vi "RemoveCaliperEntry.vi"(6 "CaliperListName":string, 7 "AnalysisResult":string[][](array[string]), 9 "CaliperList":i32, 11 "CaliperEntryList":T1[](array[typedef]) {"CaliperType" items=["Distance", "Mid Point", "Perpendicular Projection", "Lines Intersection", "Angle from Horizontal", "Angle from Vertical", "Angle Defined by 3 Points", "Angle Defined by 4 Points", "Bissecting Line", "Mid Line", "Center of Mass", "Area", "Line Fit", "Circle Fit", "Ellipse Fit"]}) -> (3 "CaliperEntryList Out":T1[](array[typedef]) {"CaliperType" items=["Distance", "Mid Point", "Perpendicular Projection", "Lines Intersection", "Angle from Horizontal", "Angle from Vertical", "Angle Defined by 3 Points", "Angle Defined by 4 Points", "Bissecting Line", "Mid Line", "Center of Mass", "Area", "Line Fit", "Circle Fit", "Ellipse Fit"]})   [LabVIEW 2019]
uses:
  Controls/CaliperDataEntry.ctl
  Controls/CaliperType.ctl
  Controls/SelectionListEntry.ctl
  Controls/SelectionListEntryPointType.ctl
  Controls/CaliperResult.ctl
panel:
  out "indexes of element":i32[](array[numeric])
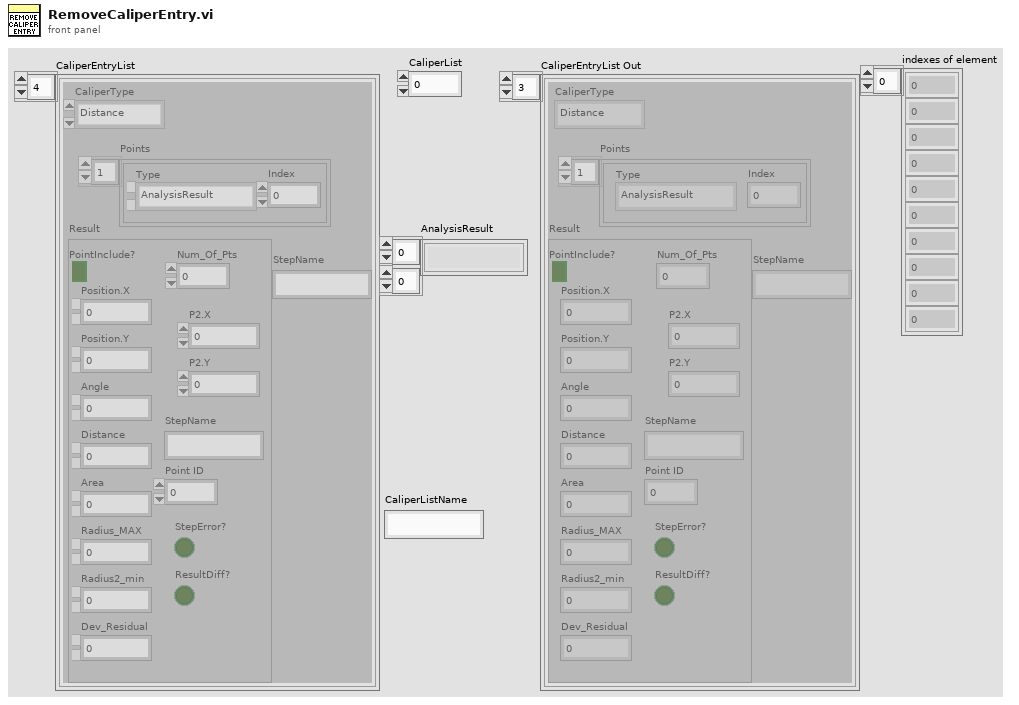
[diagram p1: front panel]
types:
  T1 = typedef "CaliperDataEntry.ctl" = cluster{"CaliperType":T2, "Points":T3[], "Result":T5, "StepName":string}
  T2 = typedef "CaliperType.ctl" = u32
  T3 = typedef "SelectionListEntry.ctl" = cluster{"Type":T4, "Index":i32}
  T4 = typedef "SelectionListEntryPointType.ctl" = enum16{"AnalysisResult", "CaliperResult"}
  T5 = typedef "CaliperResult.ctl" = cluster{"PointInclude?":bool, "Num_Of_Pts":u8, "Position.X":dbl, "Position.Y":dbl, "Angle":dbl, "Distance":dbl, "Area":dbl, "Radius_MAX":dbl, "Radius2_min":dbl, "Dev_Residual":dbl, "P2.X":dbl, "P2.Y":dbl, "StepName":string, "Point ID":u8, "StepError?":bool, "ResultDiff?":bool}
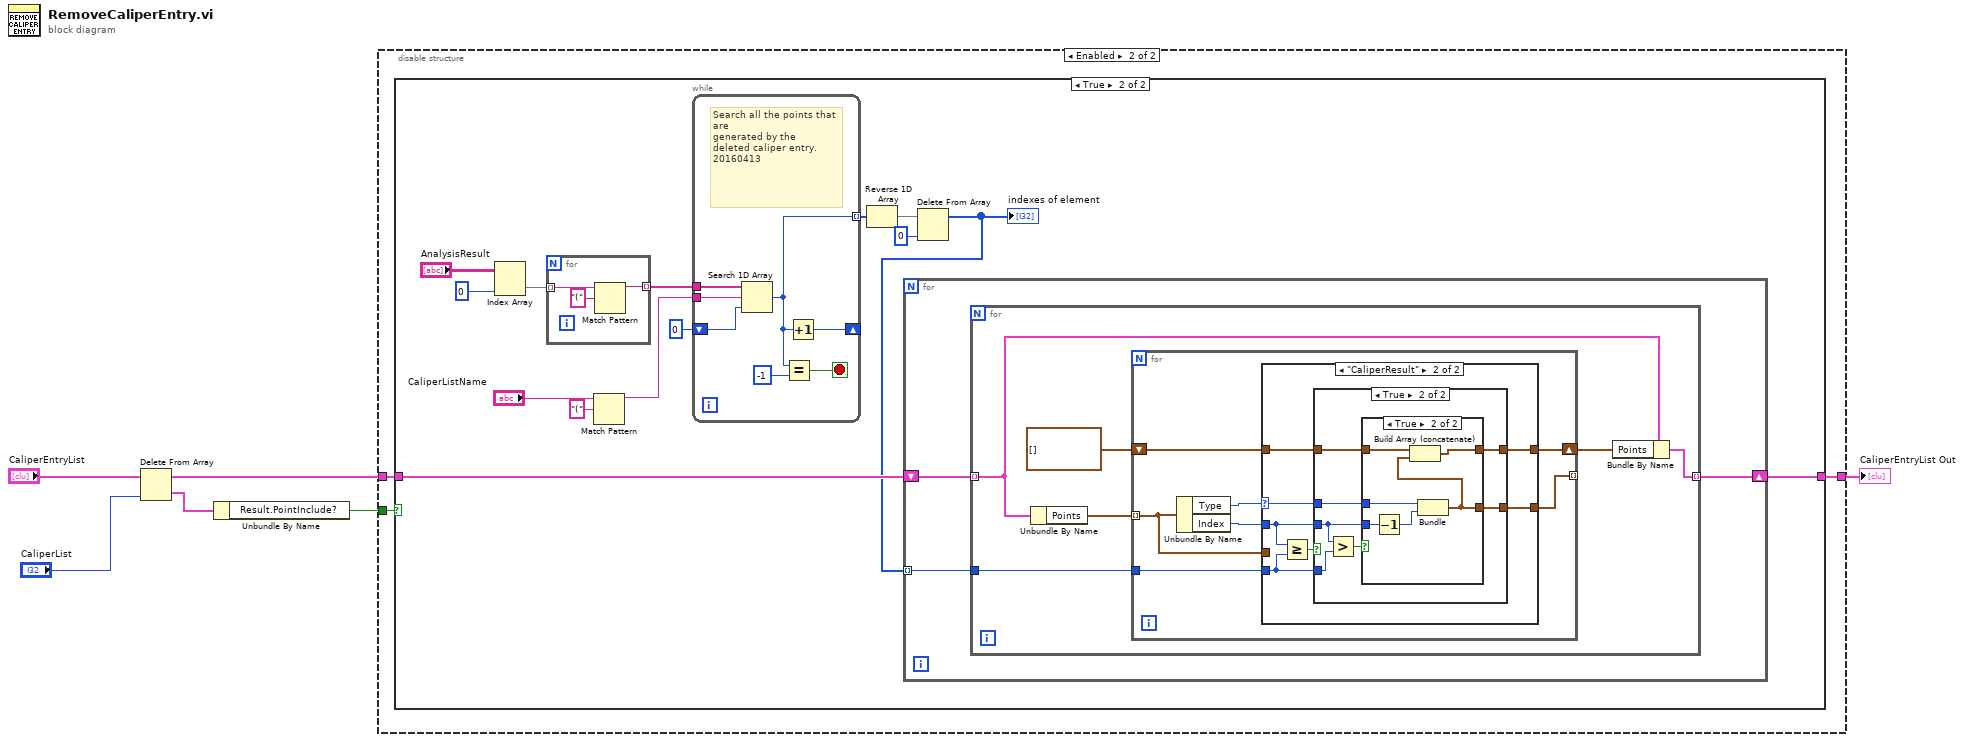
[diagram p0: block diagram]
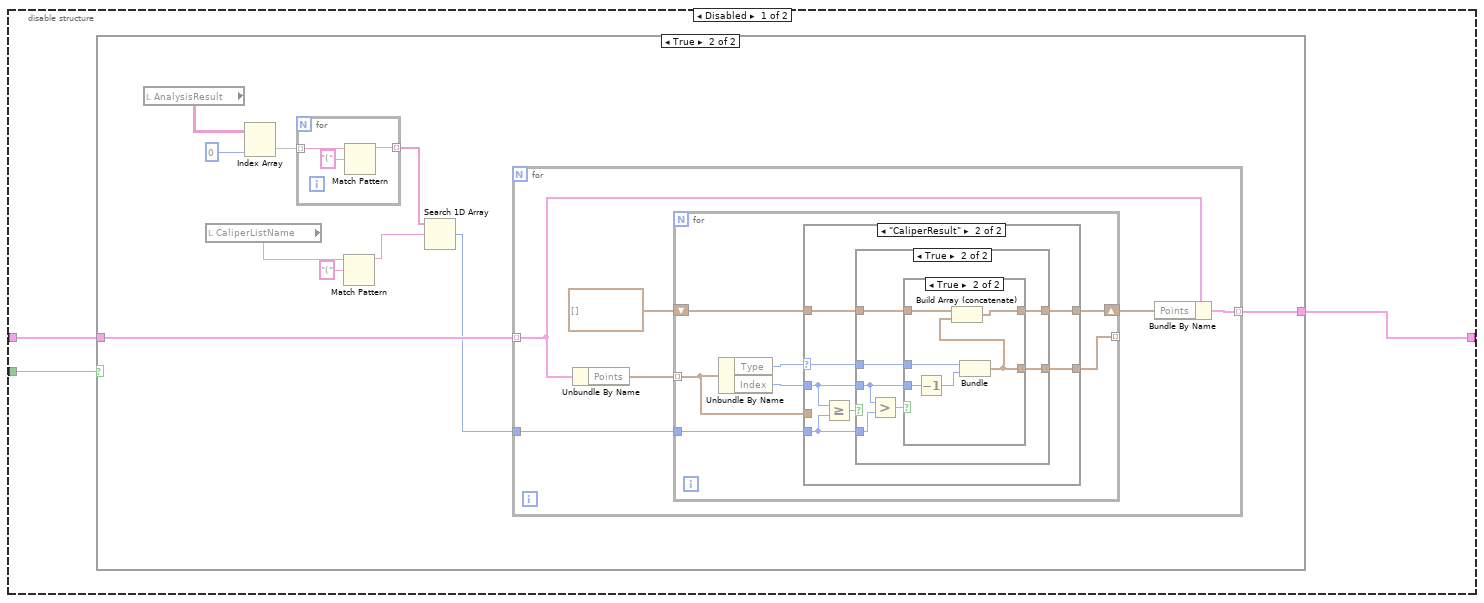
[diagram p2: hidden frame]
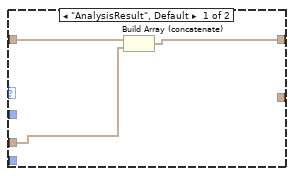
[diagram p4: hidden frame]
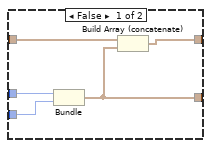
[diagram p5: hidden frame]
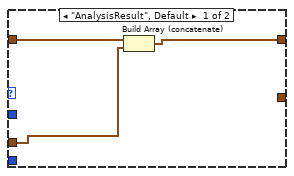
[diagram p8: hidden frame]
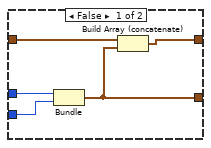
[diagram p9: hidden frame]
diagram:
  n1 = Delete From Array(array="CaliperEntryList", index="CaliperList") -> (deleted portion=w2:T1, array with subset deleted=w6:T1[])  [unwired: 1 in]
  n2 = Unbundle By Name(w2) -> ("Result.PointInclude?"=w1:bool)
  n3 = disable-structure shown="Enabled" {
    disable-tunnel: w6 -> [w9 w68]
    disable-tunnel: [w8 w67] -> w3
    disable-tunnel: w1 -> [w7 w66]
    frame Disabled {
      n4 = case shown="True" w7 {
        tunnel: w9 -> [w10 w20]
        tunnel: [w10 w19] -> w8
        frame False {
        }
        frame True {
          n5 = local read "AnalysisResult"() -> (w12:string[][])
          n6 = local read "CaliperListName"() -> (w11:string)
          n7 = Index Array(array=w12, index (col)=0 ("disabled index (col)")) -> (element=w17:string[])  [unwired: 1 in]
          n8 = for {
            tunnel: w17 -> [w23] mode=indexing
            tunnel: [w21] -> w16 mode=indexing
            n9 = Match Pattern(string=w23, regular expression="(") -> (before substring=w21:string)  [unwired: 1 in, 3 out]
          }
          n10 = Match Pattern(string=w11, regular expression="(") -> (before substring=w14:string)  [unwired: 1 in, 3 out]
          n11 = Search 1D Array(1D array=w16, element=w14) -> (index of element=w13:i32)  [unwired: 1 in]
          n12 = for {
            tunnel: w20 -> [w28] mode=indexing
            tunnel: [w27] -> w19 mode=indexing
            tunnel: w13 -> [w26]
            n13 = Unbundle By Name(w28) -> ("Points"=w29:T3[])
            n14 = for {
              tunnel: w29 -> [w34] mode=indexing
              tunnel: [w35] -> _ mode=indexing
              tunnel: w26 -> [w36]
              shift-right: [w30] -> w24
              shift-left: T3[] [] ("Points") -> [w31]
              n15 = Unbundle By Name(w34) -> ("Type"=w32:T4, "Index"=w33:i32)
              n16 = case shown="\"CaliperResult\"" w32 {
                selector: w32 -> [_ w45]
                tunnel: w34 -> [w38 _]
                tunnel: [_ w44] -> w35
                tunnel: w33 -> [_ w43]
                tunnel: w36 -> [_ w42]
                tunnel: w31 -> [w39 w41]
                tunnel: [w37 w40] -> w30
                frame "AnalysisResult", Default {
                  n17 = Build Array (concatenate)(w39, w38) -> (w37:T3[])
                }
                frame "CaliperResult" {
                  n18 = Greater Or Equal?(x=w43, y=w42) -> (x >= y?=w46:bool)
                  n19 = case shown="True" w46 {
                    tunnel: w45 -> [w51 w55]
                    tunnel: [w48 w56] -> w44
                    tunnel: w43 -> [w50 w54]
                    tunnel: w42 -> [_ w58]
                    tunnel: w41 -> [w49 w53]
                    tunnel: [w47 w52] -> w40
                    frame False {
                      n20 = Bundle("Type"=w51, "Index"=w50) -> (w48:cluster{"Type":T4, "Index":i32})  [unwired: 1 in]
                      n21 = Build Array (concatenate)(w49, w48) -> (w47:T3[])
                    }
                    frame True {
                      n22 = Greater?(x=w54, y=w58) -> (0:w57:bool)
                      n23 = case shown="True" w57 {
                        tunnel: [_ w61] -> w56
                        tunnel: w55 -> [_ w65]
                        tunnel: w54 -> [_ w64]
                        tunnel: w53 -> [w59 w62]
                        tunnel: [w59 w60] -> w52
                        frame False {
                        }
                        frame True {
                          n24 = Decrement(x=w64) -> (x-1=w63:i32)
                          n25 = Bundle("Type"=w65, w63) -> (w61:cluster{"Type":T4, i32})  [unwired: 1 in]
                          n26 = Build Array (concatenate)(w62, w61) -> (w60:T3[])
                        }
                      }
                    }
                  }
                }
              }
            }
            n27 = Bundle By Name(cluster=w28, "Points"=w24) -> (w27:T1)
          }
        }
      }
    }
    frame Enabled {
      n28 = case shown="True" w66 {
        tunnel: w68 -> [w69 w83]
        tunnel: [w69 w82] -> w67
        frame False {
        }
        frame True {
          n29 = Index Array(array="AnalysisResult", index (col)=0 ("disabled index (col)")) -> (element=w80:string[])  [unwired: 1 in]
          n30 = for {
            tunnel: w80 -> [w138] mode=indexing
            tunnel: [w136] -> w72 mode=indexing
            n31 = Match Pattern(string=w138, regular expression="(") -> (before substring=w136:string)  [unwired: 1 in, 3 out]
          }
          n32 = Match Pattern(string="CaliperListName", regular expression="(") -> (before substring=w71:string)  [unwired: 1 in, 3 out]
          n33 = while {
            tunnel: w72 -> [w135]
            tunnel: w71 -> [w134]
            tunnel: [w131] -> w76 mode=indexing
            shift-right: [w129] -> _
            shift-left: 0 ("index of element") -> [w130]
            stop <- w132 stop-if-true
            # "Search all the points that are \ngenerated by the \ndeleted caliper entry. 20160413"
            n34 = Search 1D Array(1D array=w135, element=w134, start index (0)=w130) -> (index of element=w131:i32)
            n35 = Equal?(x=w131, y=-1) -> (x = y?=w132:bool)
            n36 = Increment(x=w131) -> (x+1=w129:i32)
          }
          n37 = Reverse 1D Array(array=w76) -> (reversed array=w74:i32[])
          n38 = Delete From Array(array=w74, index=0) -> (array with subset deleted=w70:i32[])  [unwired: 1 in, 1 out]
          "indexes of element" <- w70
          n39 = for {
            shift-right: [w85] -> w82
            shift-left: w83 -> [w86]
            tunnel: w70 -> [w84] mode=indexing
            n40 = for {
              tunnel: w86 -> [w91] mode=indexing
              tunnel: [w90] -> w85 mode=indexing
              tunnel: w84 -> [w89]
              n41 = Unbundle By Name(w91) -> ("Points"=w92:T3[])
              n42 = for {
                tunnel: w92 -> [w97] mode=indexing
                tunnel: [w98] -> _ mode=indexing
                tunnel: w89 -> [w99]
                shift-right: [w93] -> w87
                shift-left: T3[] [] ("Points") -> [w94]
                n43 = Unbundle By Name(w97) -> ("Type"=w95:T4, "Index"=w96:i32)
                n44 = case shown="\"CaliperResult\"" w95 {
                  selector: w95 -> [_ w108]
                  tunnel: w97 -> [w101 _]
                  tunnel: [_ w107] -> w98
                  tunnel: w96 -> [_ w106]
                  tunnel: w99 -> [_ w105]
                  tunnel: w94 -> [w102 w104]
                  tunnel: [w100 w103] -> w93
                  frame "AnalysisResult", Default {
                    n45 = Build Array (concatenate)(w102, w101) -> (w100:T3[])
                  }
                  frame "CaliperResult" {
                    n46 = Greater Or Equal?(x=w106, y=w105) -> (x >= y?=w109:bool)
                    n47 = case shown="True" w109 {
                      tunnel: w108 -> [w114 w118]
                      tunnel: [w111 w119] -> w107
                      tunnel: w106 -> [w113 w117]
                      tunnel: w105 -> [_ w121]
                      tunnel: w104 -> [w112 w116]
                      tunnel: [w110 w115] -> w103
                      frame False {
                        n48 = Bundle("Type"=w114, "Index"=w113) -> (w111:cluster{"Type":T4, "Index":i32})  [unwired: 1 in]
                        n49 = Build Array (concatenate)(w112, w111) -> (w110:T3[])
                      }
                      frame True {
                        n50 = Greater?(x=w117, y=w121) -> (0:w120:bool)
                        n51 = case shown="True" w120 {
                          tunnel: [_ w124] -> w119
                          tunnel: w118 -> [_ w128]
                          tunnel: w117 -> [_ w127]
                          tunnel: w116 -> [w122 w125]
                          tunnel: [w122 w123] -> w115
                          frame False {
                          }
                          frame True {
                            n52 = Decrement(x=w127) -> (x-1=w126:i32)
                            n53 = Bundle("Type"=w128, w126) -> (w124:cluster{"Type":T4, i32})  [unwired: 1 in]
                            n54 = Build Array (concatenate)(w125, w124) -> (w123:T3[])
                          }
                        }
                      }
                    }
                  }
                }
              }
              n55 = Bundle By Name(cluster=w91, "Points"=w87) -> (w90:T1)
            }
          }
        }
      }
    }
  }
  "CaliperEntryList Out" <- w3
